vi "Parse and Set Program Enabled for Downlink.vi"(9 "Uplink String":string) -> (2 "Downlink String":string)   [LabVIEW 2010]
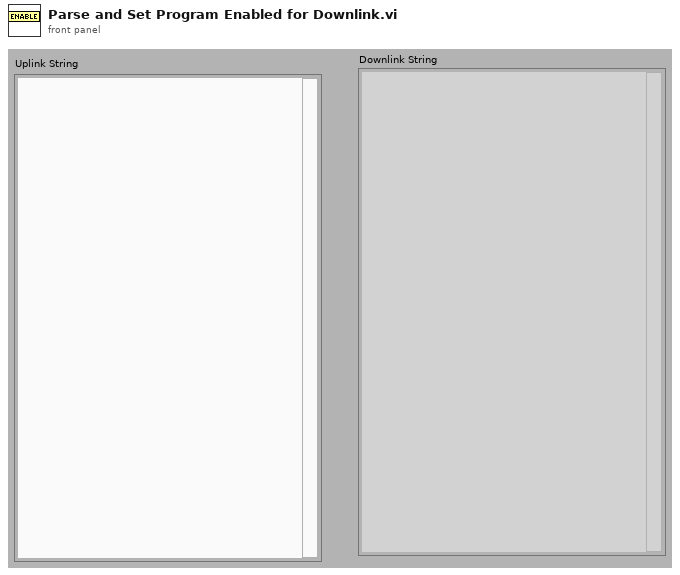
[diagram p1: front panel]
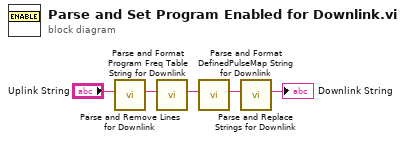
[diagram p0: block diagram]
diagram:
  n1 = call "Parse and Remove Lines for Downlink.vi"("Input String"="Uplink String") -> ("Output String"=w4:string)  [unwired: 10 in]
  n2 = call "Parse and Format Program Freq Table String for Downlink.vi"("Input String"=w4) -> ("Output String"=w3:string)  [unwired: 10 in]
  n3 = call "Parse and Format DefinedPulseMap String for Downlink.vi"("Input String"=w3) -> ("Output String"=w2:string)  [unwired: 9 in]
  n4 = call "Parse and Replace Strings for Downlink.vi"("Input String"=w2) -> ("Output String"=→"Downlink String":string)  [unwired: 9 in]
